vi "Temperatures.vi"(0 "Air Outlet Temperature (K)":dbl, 1 "Sec Cold Temp":dbl, 2 "Sec Mass Flow":dbl, 3 "Sec Hot Temp":dbl, 4 "Pri Hot Temp":dbl, 7 "Pri Cold Temp":dbl) -> (6 "Primary Hot Temperature (C)":dbl format="%#.1f", 8 "Secondary Hot Temperature (C)":dbl format="%#.1f", 9 "Primary Average Temperature (C)":dbl format="%#.1f", 10 "Secondary Cold Temperature (C)":dbl format="%#.1f", 11 "Primary Delta T (K)":dbl, 12 "Air Outlet Temperature (C)":dbl format="%#.1f", 13 "Secondary Average Temperature (C)":dbl format="%#.1f", 14 "Secondary Delta T (K)":dbl, 15 "Primary Cold Temperature (C)":dbl format="%#.1f", 16 "Secondary Average Temperature (K)":dbl, 17 "Secondary Flow (kg/s)":dbl format="%#.2f", 18 "Primary Average Temperature (K)":dbl)   [LabVIEW 2019]
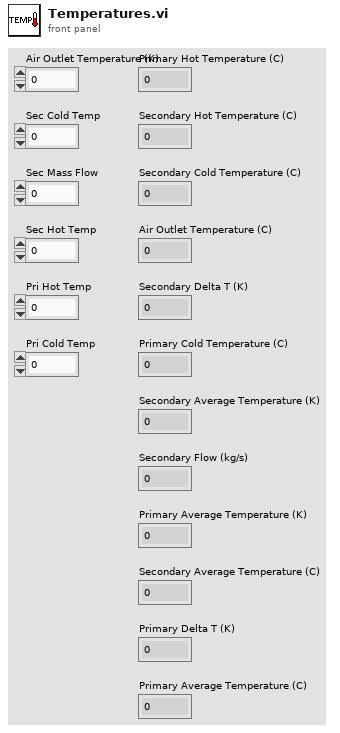
[diagram p1: front panel]
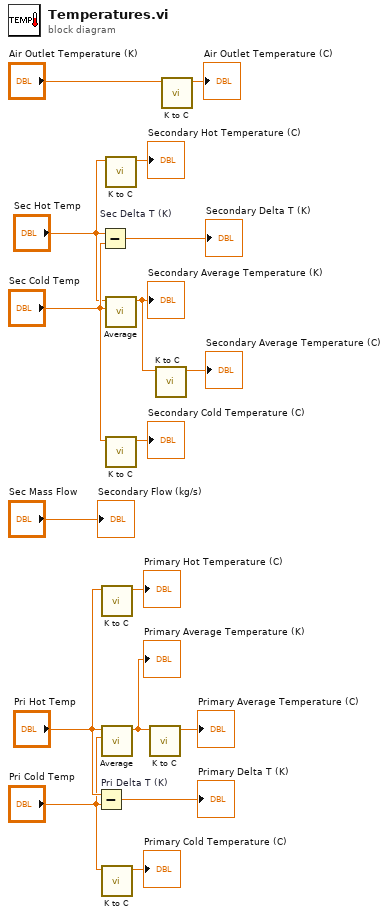
[diagram p0: block diagram]
diagram:
  n1 = Subtract "Pri Delta T (K)"(x="Pri Hot Temp", y="Pri Cold Temp") -> (x-y=→"Primary Delta T (K)":dbl)
  n2 = Subtract "Sec Delta T (K)"(x="Sec Hot Temp", y="Sec Cold Temp") -> (x-y=→"Secondary Delta T (K)":dbl)
  n3 = call "K to C.vi"("Temperature (K)"="Pri Hot Temp") -> ("Temperature (C)"=→"Primary Hot Temperature (C)":dbl)  [unwired: 10 in]
  n4 = call "Average.vi"("Number 2"="Pri Cold Temp", "Number 1"="Pri Hot Temp") -> ("Average"=w12:dbl)  [unwired: 9 in]
  "Primary Average Temperature (K)" <- w12
  n5 = call "K to C.vi"("Temperature (K)"="Pri Cold Temp") -> ("Temperature (C)"=→"Primary Cold Temperature (C)":dbl)  [unwired: 10 in]
  n6 = call "K to C.vi"("Temperature (K)"="Sec Hot Temp") -> ("Temperature (C)"=→"Secondary Hot Temperature (C)":dbl)  [unwired: 10 in]
  n7 = call "Average.vi"("Number 2"="Sec Cold Temp", "Number 1"="Sec Hot Temp") -> ("Average"=w14:dbl)  [unwired: 9 in]
  "Secondary Average Temperature (K)" <- w14
  n8 = call "K to C.vi"("Temperature (K)"="Sec Cold Temp") -> ("Temperature (C)"=→"Secondary Cold Temperature (C)":dbl)  [unwired: 10 in]
  n9 = call "K to C.vi"("Temperature (K)"=w12) -> ("Temperature (C)"=→"Primary Average Temperature (C)":dbl)  [unwired: 10 in]
  n10 = call "K to C.vi"("Temperature (K)"=w14) -> ("Temperature (C)"=→"Secondary Average Temperature (C)":dbl)  [unwired: 10 in]
  n11 = call "K to C.vi"("Temperature (K)"="Air Outlet Temperature (K)") -> ("Temperature (C)"=→"Air Outlet Temperature (C)":dbl)  [unwired: 10 in]
  "Secondary Flow (kg/s)" <- "Sec Mass Flow"
